vi "main.vi"() -> ()   [LabVIEW 2017]
uses:
  Custom_ctr/state.ctl
  <vilib>/Utility/file.llb/Write Delimited Spreadsheet (string).vi
panel:
  in  "备注内容":string
  in  "保存文件":bool
  in  "GPIB Address":u8=23
  in  "Yscale set":bool
  in  "文件保存路径":path
  out "Peak level":dbl
  out "Peak wavelength":dbl
  out "当前扫描模式":string
  in  "Log scale":dbl=10.0
  in  "Ref. Level":dbl=-20.0
  in  "Resolution":T1(ring)=enum."0.5"
  in  "Resolution set":bool
  in  "Auto Sampling":bool=TRUE
  in  "Sample PT":u16=2501 min=11 max=20001 step=1
  in  "Sens":T2(ring)=enum."Mid"
  in  "停止程序":bool
  in  "Stop sweep":bool
  in  "Repeat sweep":bool
  in  "Single sweep":bool
  in  "Sensitivity set":bool
  in  "Peak search":bool
  in  "Span set":bool
  in  "Wavelength set":bool
  out "graph":cluster{"Wavelength":sgl[], "Level":sgl[]}(graph)
  in  "Span":dbl=100.0
  in  "Center wavelength":dbl=1550.0
  in  "Stop wavelength":dbl=1600.0
  in  "Start wavelength":dbl=1500.0
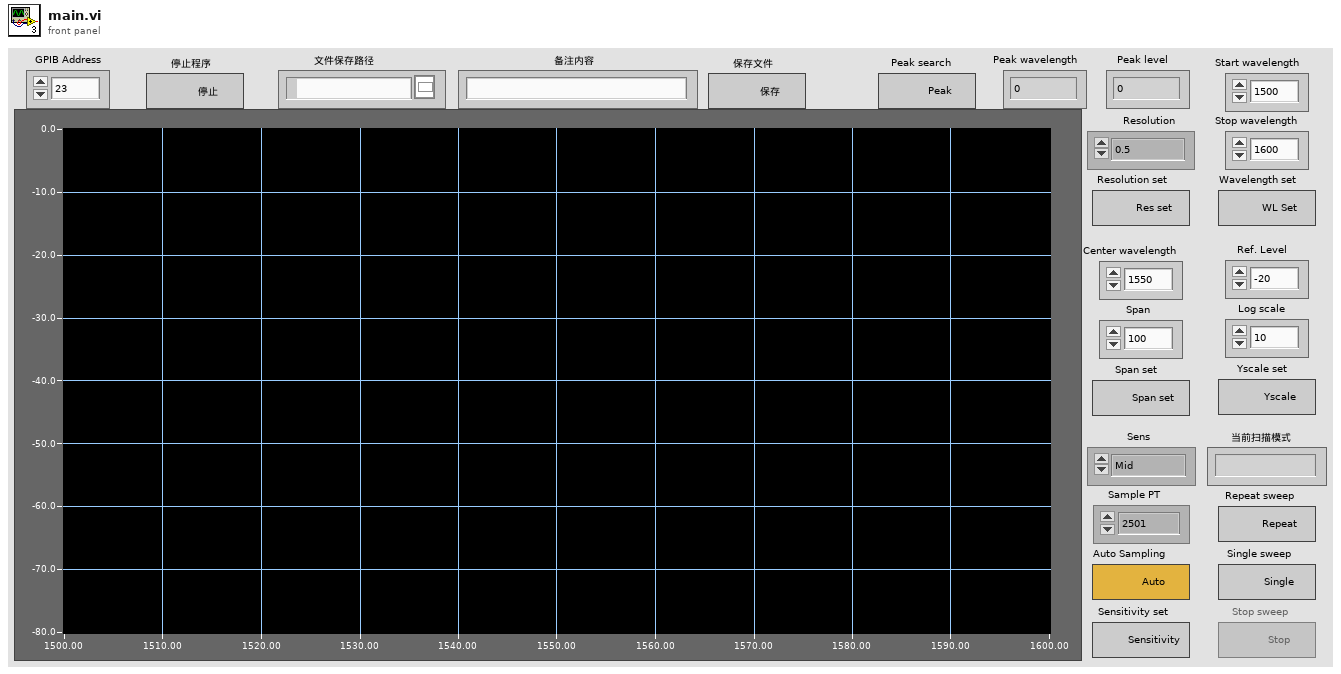
[diagram p1: front panel]
types:
  T1 = enum16{"0.01", "0.02", "0.05", "0.1", "0.2", "0.5", "1.0", "2.0"}
  T2 = enum16{"High 3", "High 2", "High 1", "Mid", "Norm Auto", "Norm Hold"}
  T3 = typedef "state.ctl" = enum16{"Initialze", "Idle", "Stop", "WL set", "Span set", "Repeat S", "Single S", "Stop S", "Sensitivity set", "Peak search", "Read trace", "Resolution set", "Yscale level"}
  T4 = enum8{"Enabled", "Disabled", "Disabled and Grayed Out"}
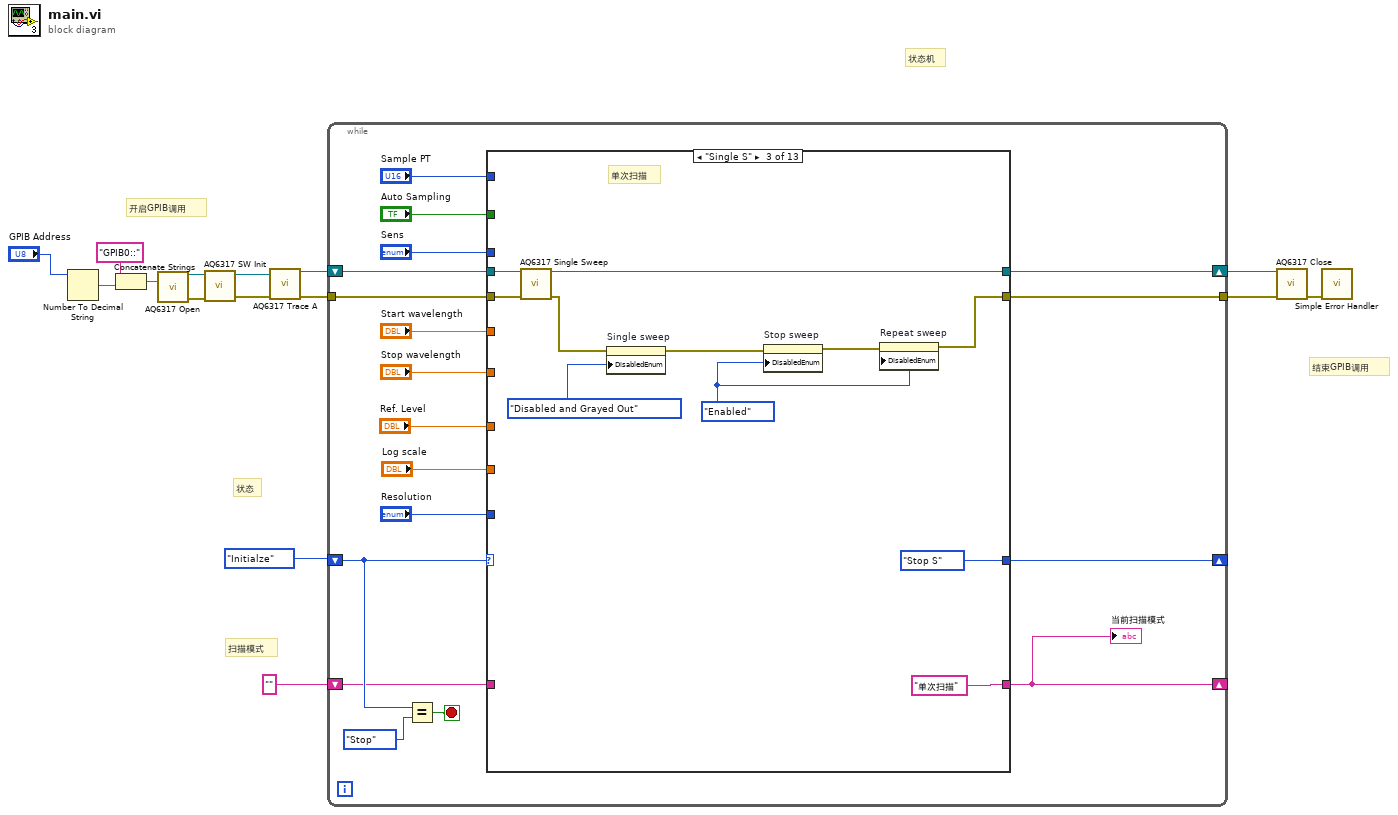
[diagram p0: block diagram]
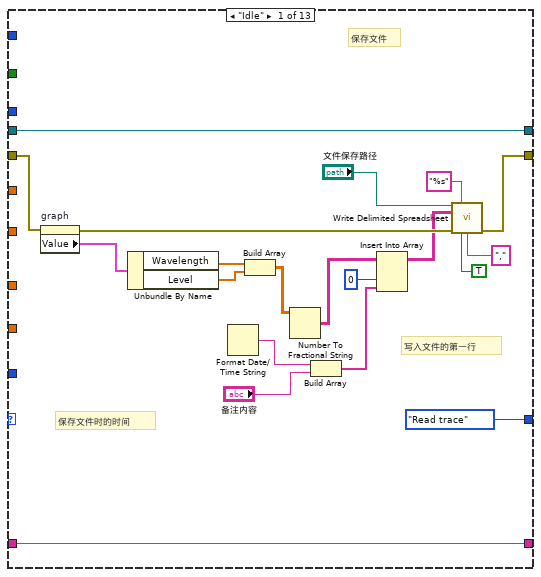
[diagram p2: hidden frame]
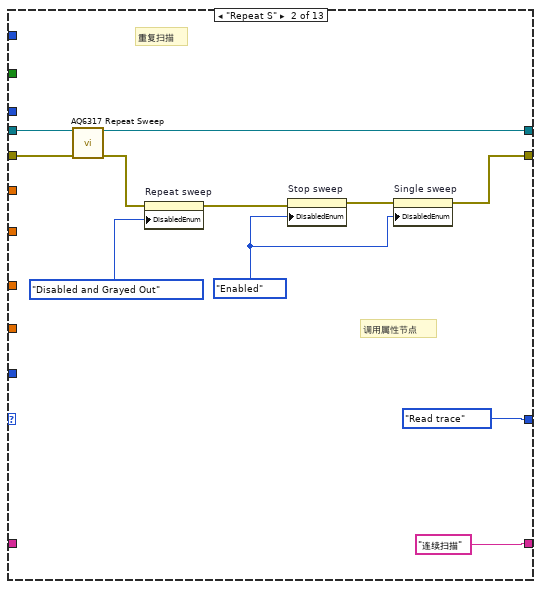
[diagram p3: hidden frame]
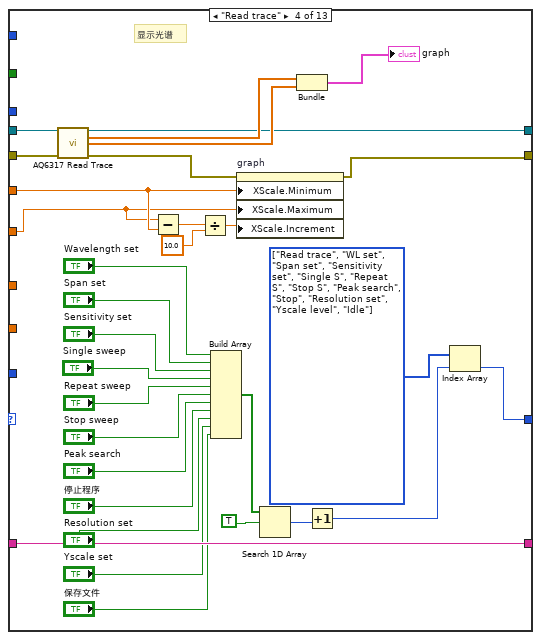
[diagram p4: hidden frame]
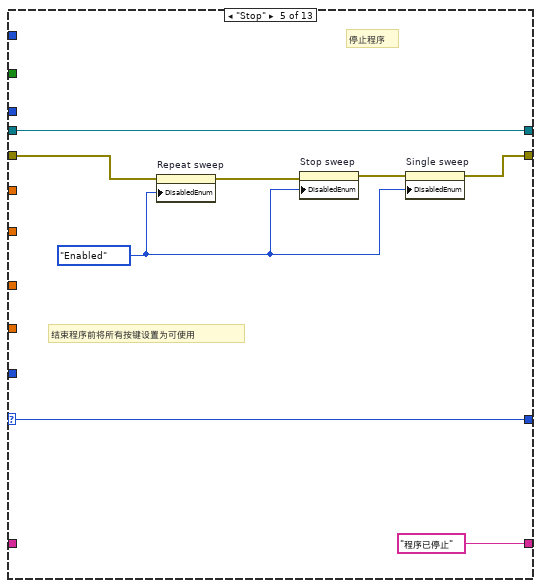
[diagram p5: hidden frame]
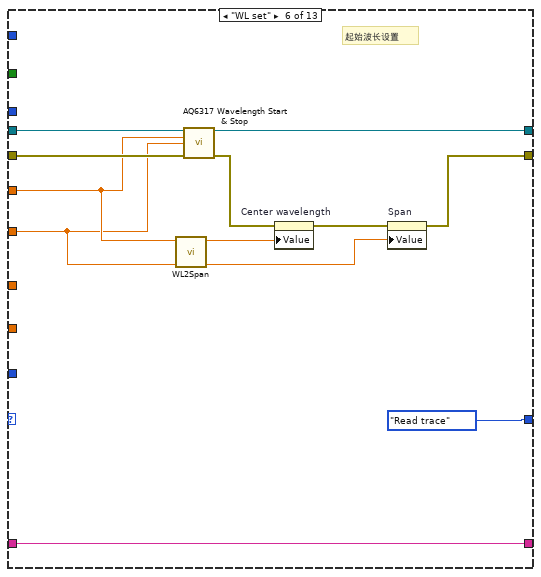
[diagram p6: hidden frame]
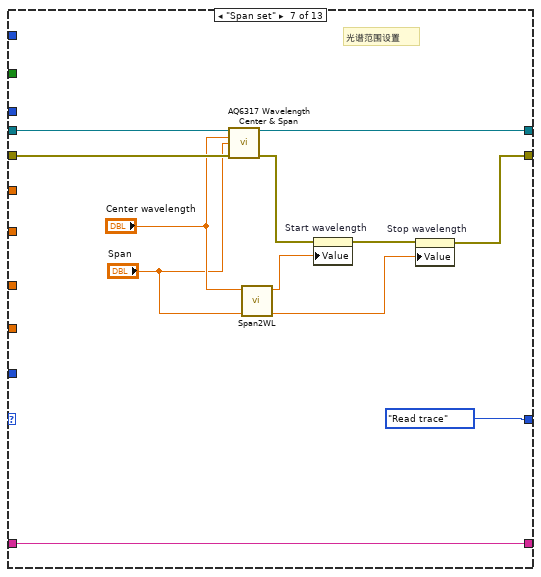
[diagram p7: hidden frame]
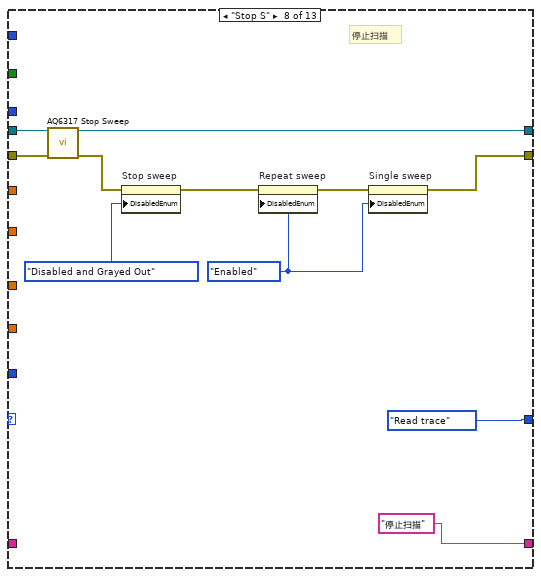
[diagram p8: hidden frame]
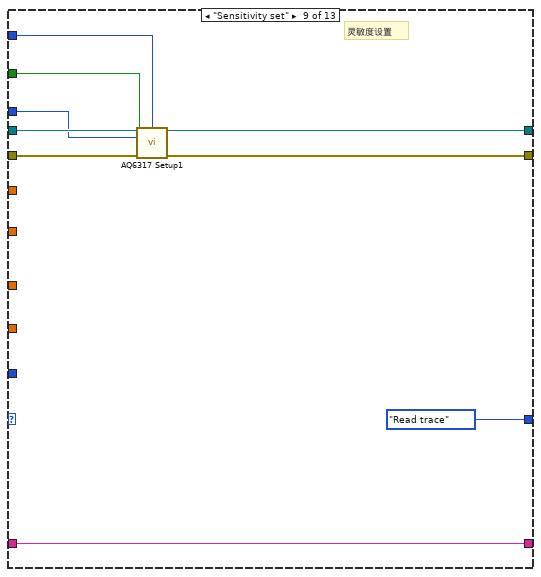
[diagram p9: hidden frame]
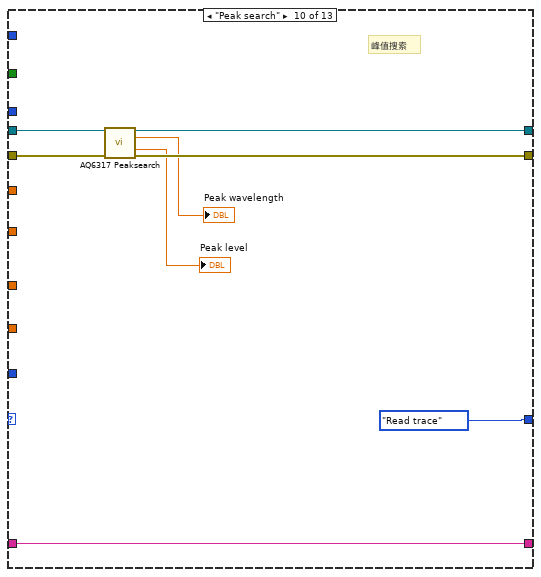
[diagram p10: hidden frame]
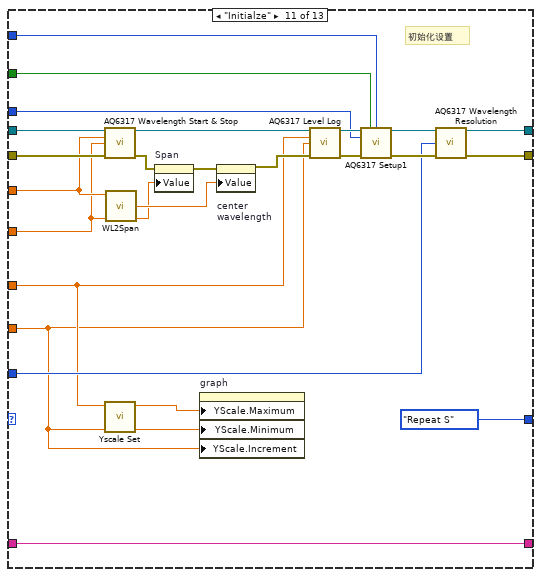
[diagram p11: hidden frame]
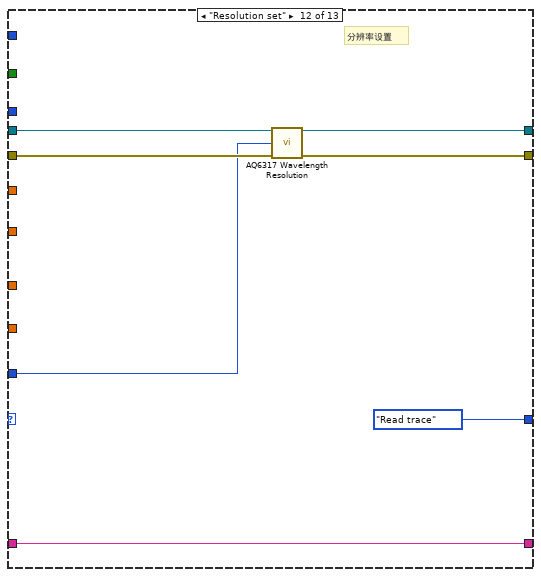
[diagram p12: hidden frame]
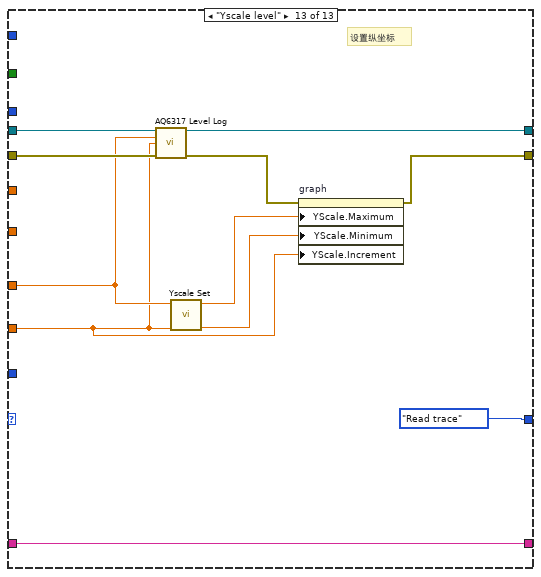
[diagram p13: hidden frame]
diagram:
  # "结束GPIB调用"
  # "状态机"
  # "开启GPIB调用"
  # "状态"
  # "扫描模式"
  n1 = Number To Decimal String(number="GPIB Address") -> (decimal integer string=w13:string)  [unwired: 1 in]
  n2 = Concatenate Strings("GPIB0::" ("Substring"), w13) -> (w11:string)
  n3 = call "AQ6317 Open.vi"("resource name (\"GPIB0::1\")"=w11) -> ("VISA session out"=w15:refnum<visa-resource-name>, "Error Out"=w14:errorcluster)  [unwired: 13 in]
  n4 = call "AQ6317 SW Init.vi"("Error In"=w14, "VISA session"=w15) -> ("Error Out"=w4:errorcluster, "dup VISA session"=w6:refnum<visa-resource-name>)  [unwired: 6 in]
  n5 = call "AQ6317 Trace A.vi"("VISA session"=w6, "Error In"=w4) -> ("dup VISA session"=w5:refnum<visa-resource-name>, "Error Out"=w3:errorcluster)  [unwired: 12 in]
  n6 = while {
    tunnel: w3 -> [w32]
    tunnel: [w31] -> w8
    shift-right: [w33] -> w9
    shift-left: w5 -> [w30]
    shift-right: [w29] -> _
    shift-left: state."Initialze" ("state") -> [w28]
    shift-right: [w17] -> _
    shift-left: "" ("当前扫描模式 2") -> [w16]
    stop <- w27 stop-if-true
    n7 = Equal?(x=w28, y=state."Stop" ("state")) -> (x = y?=w27:bool)
    n8 = case shown="\"Single S\"" w28 {
      tunnel: w30 -> [w53 w64 w75 w106 w113 w126 w138 w144 w158 w166 w192 w199 w210]
      tunnel: [w53 w63 w73 w102 w113 w124 w136 w143 w157 w163 w173 w197 w208] -> w33
      tunnel: w32 -> [w47 w62 w74 w105 w109 w125 w137 w142 w156 w165 w191 w198 w209]
      tunnel: [w49 w55 w67 w83 w108 w121 w133 w141 w155 w164 w172 w196 w202] -> w31
      selector: w28 -> [_ _ _ _ w112 _ _ _ _ _ _ _ _]
      tunnel: [state."Read trace" ("state") state."Read trace" ("state") state."Stop S" ("state") w87 w112 state."Read trace" ("state") state."Read trace" ("state") state."Read trace" ("state") state."Read trace" ("state") state."Read trace" ("state") state."Repeat S" ("state") state."Read trace" ("state") state."Read trace" ("state")] -> w29
      tunnel: "Stop wavelength" -> [_ _ _ w79 _ w117 _ _ _ _ w184 _ _]
      tunnel: "Start wavelength" -> [_ _ _ w80 _ w118 _ _ _ _ w185 _ _]
      tunnel: "Resolution" -> [_ _ _ _ _ _ _ _ _ _ w175 w194 _]
      tunnel: "Auto Sampling" -> [_ _ _ _ _ _ _ _ w154 _ w177 _ _]
      tunnel: "Sample PT" -> [_ _ _ _ _ _ _ _ w153 _ w178 _ _]
      tunnel: "Sens" -> [_ _ _ _ _ _ _ _ w152 _ w176 _ _]
      tunnel: "Ref. Level" -> [_ _ _ _ _ _ _ _ _ _ w169 _ w207]
      tunnel: "Log scale" -> [_ _ _ _ _ _ _ _ _ _ w168 _ w204]
      tunnel: [w52 "连续扫描" ("当前扫描模式 2") "单次扫描" ("当前扫描模式 2") w85 "程序已停止" ("当前扫描模式 2") w120 w132 "停止扫描" ("当前扫描模式 2") w151 w162 w167 w193 w201] -> w17
      tunnel: w16 -> [w52 _ _ w85 _ w120 w132 _ w151 w162 w167 w193 w201]
      frame "Idle" {
        # "保存文件"
        # "写入文件的第一行"
        # "保存文件时的时间"
        n9 = property on="graph" class="XYGraph (严格)"(error in=w47) -> (error out=w46:errorcluster, "Value"=w48:cluster{"Wavelength":sgl[], "Level":sgl[]})  [unwired: 1 in, 1 out]
        n10 = Unbundle By Name(w48) -> ("Wavelength"=w43:sgl[], "Level"=w45:sgl[])
        n11 = Format Date/Time String() -> (date/time string=w37:string)  [unwired: 3 in]
        n12 = Build Array(w43, w45) -> (w41:sgl[][])
        n13 = Number To Fractional String(number=w41) -> (F-format string=w35:string[][])  [unwired: 3 in]
        n14 = Build Array(w37, "备注内容") -> (w36:string[])
        n15 = Insert Into Array(array=w35, index (col)=0 ("索引 (行)"), new element=w36) -> (w40:string[][])  [unwired: 1 in]
        n16 = call-poly <vilib>:"Write Delimited Spreadsheet.vi"("file path (dialog if empty)"="文件保存路径", "format (%s)"="%s", "2D data"=w40, "error in (no error)"=w46, "transpose? (no:F)"=TRUE, "delimiter (\\t)"="," ("delimiter (\\t)")) -> ("error out"=w49:errorcluster)  [unwired: 8 in, 1 out]
      }
      frame "Repeat S" {
        w59 = T4."Enabled" ("禁用")
        # "重复扫描"
        # "调用属性节点"
        n17 = call "AQ6317 Repeat Sweep.vi"("VISA session"=w64, "Error In"=w62) -> ("dup VISA session"=w63:refnum<visa-resource-name>, "Error Out"=w58:errorcluster)  [unwired: 12 in]
        n18 = property on="Repeat sweep" class="Bool"(error in=w58, "DisabledEnum"=T4."Disabled and Grayed Out" ("禁用")) -> (error out=w57:errorcluster)  [unwired: 1 in, 1 out]
        n19 = property on="Stop sweep" class="Bool"(error in=w57, "DisabledEnum"=w59) -> (error out=w56:errorcluster)  [unwired: 1 in, 1 out]
        n20 = property on="Single sweep" class="Bool"(error in=w56, "DisabledEnum"=w59) -> (error out=w55:errorcluster)  [unwired: 1 in, 1 out]
      }
      frame "Single S" {
        w71 = T4."Enabled" ("禁用")
        # "单次扫描"
        n21 = call "AQ6317 Single Sweep.vi"("VISA session"=w75, "Error In"=w74) -> ("dup VISA session"=w73:refnum<visa-resource-name>, "Error Out"=w68:errorcluster)  [unwired: 12 in]
        n22 = property on="Single sweep" class="Bool"(error in=w68, "DisabledEnum"=T4."Disabled and Grayed Out" ("禁用")) -> (error out=w70:errorcluster)  [unwired: 1 in, 1 out]
        n23 = property on="Stop sweep" class="Bool"(error in=w70, "DisabledEnum"=w71) -> (error out=w69:errorcluster)  [unwired: 1 in, 1 out]
        n24 = property on="Repeat sweep" class="Bool"(error in=w69, "DisabledEnum"=w71) -> (error out=w67:errorcluster)  [unwired: 1 in, 1 out]
      }
      frame "Read trace" {
        w90 = T3[] [enum."Read trace", enum."WL set", enum."Span set", enum."Sensitivity set", enum."Single S", enum."Repeat S", enum."Stop S", enum."Peak search", enum."Stop", enum."Resolution set", enum."Yscale level", enum."Idle"] items=["Initialze", "Idle", "Stop", "WL set", "Span set", "Repeat S", "Single S", "Stop S", "Sensitivity set", "Peak search", "Read trace", "Resolution set", "Yscale level"]
        # "显示光谱"
        n25 = call "AQ6317 Read Trace.vi"("VISA session"=w106, "Error In"=w105) -> ("dup VISA session"=w102:refnum<visa-resource-name>, "Wavelength"=w104:sgl[], "Level"=w103:sgl[], "Error Out"=w84:errorcluster)  [unwired: 8 in, 2 out]
        n26 = Subtract(x=w79, y=w80) -> (x-y=w81:dbl)
        n27 = Divide(x=w81, y=10.0) -> (x/y=w82:dbl)
        n28 = Build Array("Wavelength set", "Span set", "Sensitivity set", "Single sweep", "Repeat sweep", "Stop sweep", "Peak search", "停止程序", "Resolution set", "Yscale set", "保存文件") -> (w101:bool[])
        n29 = property on="graph" class="XYGraph (严格)"(error in=w84, "XScale.Minimum"=w80, "XScale.Maximum"=w79, "XScale.Increment"=w82) -> (error out=w83:errorcluster)  [unwired: 1 in, 1 out]
        n30 = Search 1D Array(1D array=w101, element=TRUE) -> (index of element=w97:i32)  [unwired: 1 in]
        n31 = Bundle("Wavelength"=w104, "Level"=w103) -> (→"graph":cluster{"Wavelength":sgl[], "Level":sgl[]})  [unwired: 1 in]
        n32 = Increment(x=w97) -> (x+1=w98:i32)
        n33 = Index Array(array=w90, index=w98) -> (element=w87:T3)
      }
      frame "Stop" {
        w107 = T4."Enabled" ("禁用")
        # "结束程序前将所有按键设置为可使用"
        # "停止程序"
        n34 = property on="Repeat sweep" class="Bool"(error in=w109, "DisabledEnum"=w107) -> (error out=w111:errorcluster)  [unwired: 1 in, 1 out]
        n35 = property on="Stop sweep" class="Bool"(error in=w111, "DisabledEnum"=w107) -> (error out=w110:errorcluster)  [unwired: 1 in, 1 out]
        n36 = property on="Single sweep" class="Bool"(error in=w110, "DisabledEnum"=w107) -> (error out=w108:errorcluster)  [unwired: 1 in, 1 out]
      }
      frame "WL set" {
        # "起始波长设置"
        n37 = call "WL2Span.vi"("stop"=w117, "start"=w118) -> ("span"=w115:dbl, "center"=w116:dbl)  [unwired: 8 in]
        n38 = call "AQ6317 Wavelength Start & Stop.vi"("VISA session"=w126, "Start (750 nm)"=w118, "Stop (1750 nm)"=w117, "Error In"=w125) -> ("dup VISA session"=w124:refnum<visa-resource-name>, "Error Out"=w123:errorcluster)  [unwired: 10 in]
        n39 = property on="Center wavelength" class="DigNum (严格)"(error in=w123, "Value"=w116) -> (error out=w122:errorcluster)  [unwired: 1 in, 1 out]
        n40 = property on="Span" class="DigNum (严格)"(error in=w122, "Value"=w115) -> (error out=w121:errorcluster)  [unwired: 1 in, 1 out]
      }
      frame "Span set" {
        # "光谱范围设置"
        n41 = call "AQ6317 Wavelength Center & Span.vi"("VISA session"=w138, "Center (1250 nm)"="Center wavelength", "Span (1000 nm)"="Span", "Error In"=w137) -> ("dup VISA session"=w136:refnum<visa-resource-name>, "Error Out"=w135:errorcluster)  [unwired: 10 in]
        n42 = call "Span2WL.vi"("span"="Span", "center"="Center wavelength") -> ("stop"=w127:dbl, "start"=w128:dbl)  [unwired: 8 in]
        n43 = property on="Start wavelength" class="DigNum (严格)"(error in=w135, "Value"=w128) -> (error out=w134:errorcluster)  [unwired: 1 in, 1 out]
        n44 = property on="Stop wavelength" class="DigNum (严格)"(error in=w134, "Value"=w127) -> (error out=w133:errorcluster)  [unwired: 1 in, 1 out]
      }
      frame "Stop S" {
        w145 = T4."Enabled" ("禁用")
        # "停止扫描"
        n45 = call "AQ6317 Stop Sweep.vi"("VISA session"=w144, "Error In"=w142) -> ("dup VISA session"=w143:refnum<visa-resource-name>, "Error Out"=w149:errorcluster)  [unwired: 12 in]
        n46 = property on="Stop sweep" class="Bool"(error in=w149, "DisabledEnum"=T4."Disabled and Grayed Out" ("禁用")) -> (error out=w148:errorcluster)  [unwired: 1 in, 1 out]
        n47 = property on="Repeat sweep" class="Bool"(error in=w148, "DisabledEnum"=w145) -> (error out=w147:errorcluster)  [unwired: 1 in, 1 out]
        n48 = property on="Single sweep" class="Bool"(error in=w147, "DisabledEnum"=w145) -> (error out=w141:errorcluster)  [unwired: 1 in, 1 out]
      }
      frame "Sensitivity set" {
        # "灵敏度设置"
        n49 = call "AQ6317 Setup1.vi"("VISA session"=w158, "Auto Sampling (T)"=w154, "Sample PT(2501)"=w153, "Sens (5:Norm Hold)"=w152, "Error In"=w156) -> ("dup VISA session"=w157:refnum<visa-resource-name>, "Error Out"=w155:errorcluster)  [unwired: 9 in]
      }
      frame "Peak search" {
        # "峰值搜索"
        n50 = call "AQ6317 Peaksearch.vi"("VISA session"=w166, "Error in"=w165) -> ("dup VISA session"=w163:refnum<visa-resource-name>, "Wavelength"=→"Peak wavelength":dbl, "Level"=→"Peak level":dbl, "Error out"=w164:errorcluster)  [unwired: 9 in, 1 out]
      }
      frame "Initialze" {
        # "初始化设置"
        n51 = call "AQ6317 Wavelength Start & Stop.vi"("VISA session"=w192, "Start (750 nm)"=w185, "Stop (1750 nm)"=w184, "Error In"=w191) -> ("dup VISA session"=w190:refnum<visa-resource-name>, "Error Out"=w180:errorcluster)  [unwired: 10 in]
        n52 = call "Yscale Set.vi"("Log scale"=w168, "Ref. Level"=w169) -> ("Y min"=w170:dbl, "Y max"=w171:dbl)  [unwired: 8 in]
        n53 = call "WL2Span.vi"("stop"=w184, "start"=w185) -> ("span"=w182:dbl, "center"=w183:dbl)  [unwired: 8 in]
        n54 = property on="Span" class="DigNum (严格)"(error in=w180, "Value"=w182) -> (error out=w181:errorcluster)  [unwired: 1 in, 1 out]
        n55 = property on="graph" class="XYGraph (严格)"("YScale.Maximum"=w171, "YScale.Minimum"=w170, "YScale.Increment"=w168) -> ()  [unwired: 2 in, 2 out]
        n56 = property on="center \nwavelength" class="DigNum (严格)"(error in=w181, "Value"=w183) -> (error out=w179:errorcluster)  [unwired: 1 in, 1 out]
        n57 = call "AQ6317 Level Log.vi"("VISA session"=w190, "Ref Level dBm (0)"=w169, "Log Scale dB/D (5)"=w168, "Error in"=w179) -> ("dup VISA session"=w189:refnum<visa-resource-name>, "Error out"=w188:errorcluster)  [unwired: 10 in]
        n58 = call "AQ6317 Setup1.vi"("VISA session"=w189, "Auto Sampling (T)"=w177, "Sample PT(2501)"=w178, "Sens (5:Norm Hold)"=w176, "Error In"=w188) -> ("dup VISA session"=w187:refnum<visa-resource-name>, "Error Out"=w186:errorcluster)  [unwired: 9 in]
        n59 = call "AQ6317 Wavelength Resolution.vi"("VISA session"=w187, "Resolution (7: 2.0 nm)"=w175, "Error In"=w186) -> ("dup VISA session"=w173:refnum<visa-resource-name>, "Error Out"=w172:errorcluster)  [unwired: 11 in]
      }
      frame "Resolution set" {
        # "分辨率设置"
        n60 = call "AQ6317 Wavelength Resolution.vi"("VISA session"=w199, "Resolution (7: 2.0 nm)"=w194, "Error In"=w198) -> ("dup VISA session"=w197:refnum<visa-resource-name>, "Error Out"=w196:errorcluster)  [unwired: 11 in]
      }
      frame "Yscale level" {
        # "设置纵坐标"
        n61 = call "AQ6317 Level Log.vi"("VISA session"=w210, "Ref Level dBm (0)"=w207, "Log Scale dB/D (5)"=w204, "Error in"=w209) -> ("dup VISA session"=w208:refnum<visa-resource-name>, "Error out"=w203:errorcluster)  [unwired: 10 in]
        n62 = call "Yscale Set.vi"("Log scale"=w204, "Ref. Level"=w207) -> ("Y min"=w205:dbl, "Y max"=w206:dbl)  [unwired: 8 in]
        n63 = property on="graph" class="XYGraph (严格)"(error in=w203, "YScale.Maximum"=w206, "YScale.Minimum"=w205, "YScale.Increment"=w204) -> (error out=w202:errorcluster)  [unwired: 1 in, 1 out]
      }
    }
    "当前扫描模式" <- w17
  }
  n64 = call "AQ6317 Close.vi"("VISA session"=w9, "error in"=w8) -> ("error out"=w10:errorcluster)  [unwired: 11 in, 2 out]
  n65 = call <vilib>:"Simple Error Handler.vi"("error in (no error)"=w10) -> ()  [unwired: 4 in, 5 out]
